vi "Generic_AR.vi"() -> ()   [LabVIEW 2018]
panel:
  in  "stop":bool
  out "Graph":u16[][](graph)
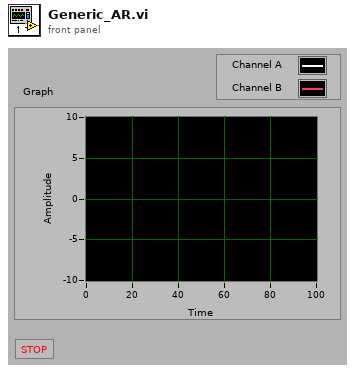
[diagram p1: front panel]
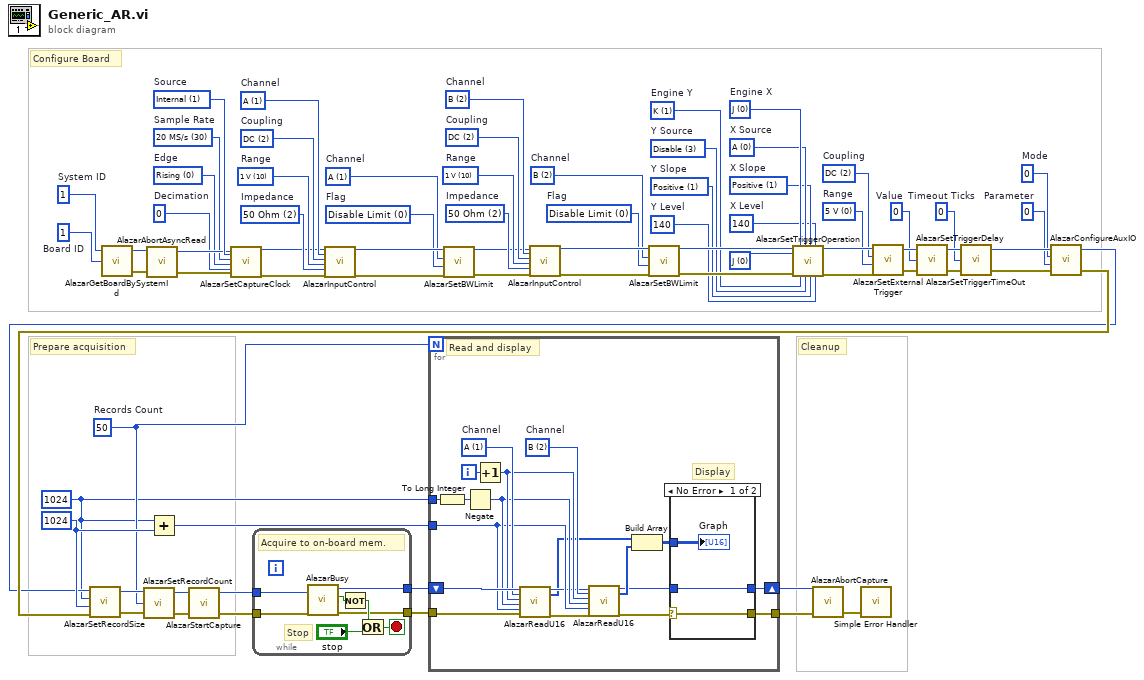
[diagram p0: block diagram]
diagram:
  w6 = u32 50  # Records Count
  w17 = u32 1024 ("Post-trigger Samples")
  w5 = u32 1024 ("Pre-trigger Samples")
  w47 = u32 0 items=["Disable Limit", "Enable Limit"]  # Flag
  w46 = u32 2 items=["A"=1, "B"=2, "C"=4, "D"=8]  # Channel
  w50 = u32 2 items=["1 MOhm"=1, "50 Ohm"=2]  # Impedance
  w44 = u32 10 items=["20 mV"=1, "40 mV"=2, "50 mV"=3, "80 mV"=4, "100 mV"=5, "200 mV"=6, "400 mV"=7, "500 mV"=8, "800 mV"=9, "1 V"=10, "1.25 V"=33, "2 V"=11, "4 V"=12, "5 V"=13, "8 V"=14, "10 V"=15, "20 V"=16]  # Range
  w51 = u32 2 items=["AC"=1, "DC"=2]  # Coupling
  w52 = u8 2 items=["A"=1, "B"=2, "C"=4, "D"=8]  # Channel
  w20 = u32 0  # Parameter
  w19 = u32 0  # Mode
  w18 = u32 0  # Timeout Ticks
  w25 = u32 0  # Value
  w29 = u32 0 items=["5 V", "1 V", "TTL"]  # Range
  w28 = u32 2 items=["AC"=1, "DC"=2]  # Coupling
  w32 = u32 140  # Y Level
  w33 = u32 1 items=["Positive"=1, "Negative"=2]  # Y Slope
  w34 = u32 3 items=["A", "B", "External", "Disable", "C", "D"]  # Y Source
  w36 = u32 140  # X Level
  w37 = u32 1 items=["Positive"=1, "Negative"=2]  # X Slope
  w38 = u32 0 items=["A", "B", "External", "Disable", "C", "D"]  # X Source
  w35 = u32 1 items=["J", "K"]  # Engine Y
  w39 = u32 0 items=["J", "K"]  # Engine X
  w40 = u32 0 items=["J", "K", "J OR K", "J AND K", "J XOR K", "J AND NOT K", "NOT J AND K"] ("Op.")
  w54 = u32 0 items=["Disable Limit", "Enable Limit"]  # Flag
  w53 = u32 1 items=["A"=1, "B"=2, "C"=4, "D"=8]  # Channel
  w59 = u32 2 items=["1 MOhm"=1, "50 Ohm"=2]  # Impedance
  w60 = u32 10 items=["20 mV"=1, "40 mV"=2, "50 mV"=3, "80 mV"=4, "100 mV"=5, "200 mV"=6, "400 mV"=7, "500 mV"=8, "800 mV"=9, "1 V"=10, "1.25 V"=33, "2 V"=11, "4 V"=12, "5 V"=13, "8 V"=14, "10 V"=15, "20 V"=16]  # Range
  w61 = u32 2 items=["AC"=1, "DC"=2]  # Coupling
  w62 = u8 1 items=["A"=1, "B"=2, "C"=4, "D"=8]  # Channel
  w64 = u32 0  # Decimation
  w65 = u32 0 items=["Rising", "Falling"]  # Edge
  w66 = u32 30 items=["1 kS/s"=1, "2 kS/s"=2, "5 kS/s"=4, "10 kS/s"=8, "20 kS/s"=10, "50 kS/s"=12, "100 kS/s"=14, "200 kS/s"=16, "500 kS/s"=18, "1 MS/s"=20, "2 MS/s"=24, "5 MS/s"=26, "10 MS/s"=28, "20 MS/s"=30, "25 MS/s"=33, "50 MS/s"=34, "100 MS/s"=36, "125 MS/s"=37, "160 MS/s"=38, "180 MS/s"=39, "250 MS/s"=43, "500 MS/s"=48, "800 MS/s"=50, "1000 MS/s"=53, "1200 MS/s"=55, "1500 MS/s"=58, "1800 MS/s"=61, "USER_DEF"=0]  # Sample Rate
  w68 = u32 1 items=["Internal"=1, "External"=2]  # Source
  w72 = u32 1  # Board ID
  w71 = u32 1  # System ID
  # "Cleanup"
  # "Prepare acquisition"
  # "Configure Board"
  n1 = call "AlazarGetBoardBySystemId.vi"("Board ID"=w72, "System ID"=w71) -> ("error out"=w69:errorcluster, "Handle"=w70:u64)  [unwired: 1 in, 1 out]
  n2 = call "AlazarAbortAsyncRead.vi"("Handle"=w70, "error in (no error)"=w69) -> ("Handle"=w67:u64, "error out"=w63:errorcluster)  [unwired: 1 out]
  n3 = Add(x=w5, y=w17) -> (x+y=w4:u32)
  n4 = call "AlazarSetCaptureClock.vi"("Handle"=w67, "Source"=w68, "Sample Rate"=w66, "Edge"=w65, "Decimation"=w64, "error in (no error)"=w63) -> ("Handle"=w58:u64, "error out"=w57:errorcluster)  [unwired: 11 in, 1 out]
  n5 = call "AlazarInputControl.vi"("Handle"=w58, "Channel"=w62, "Coupling"=w61, "Range"=w60, "Impedance"=w59, "error in (no error)"=w57) -> ("Handle"=w56:u64, "error out"=w55:errorcluster)  [unwired: 11 in, 1 out]
  n6 = call "AlazarSetBWLimit.vi"("error in (no error)"=w55, "Flag"=w54, "Channel"=w53, "Handle"=w56) -> ("error out"=w45:errorcluster, "Handle"=w43:u64)  [unwired: 1 out]
  n7 = call "AlazarInputControl.vi"("Handle"=w43, "Channel"=w52, "Coupling"=w51, "Range"=w44, "Impedance"=w50, "error in (no error)"=w45) -> ("Handle"=w49:u64, "error out"=w48:errorcluster)  [unwired: 11 in, 1 out]
  n8 = call "AlazarSetBWLimit.vi"("error in (no error)"=w48, "Flag"=w47, "Channel"=w46, "Handle"=w49) -> ("error out"=w41:errorcluster, "Handle"=w42:u64)  [unwired: 1 out]
  n9 = call "AlazarSetTriggerOperation.vi"("Handle"=w42, "Trigger Operation"=w40, "error in (no error)"=w41, "Trigger Engine 1"=w39, "Trigger Engine 2"=w35, "Source 1"=w38, "Source 2"=w34, "Slope 1"=w37, "Slope 2"=w33, "Level 1"=w36, "Level 2"=w32) -> ("Handle"=w31:u64, "error out"=w30:errorcluster)  [unwired: 6 in, 1 out]
  n10 = call "AlazarSetExternalTrigger.vi"("error in (no error)"=w30, "Range ID"=w29, "Coupling ID"=w28, "Handle"=w31) -> ("error out"=w26:errorcluster, "Handle"=w27:u64)  [unwired: 1 out]
  n11 = call "AlazarSetTriggerDelay.vi"("error in (no error)"=w26, "Delay"=w25, "Handle"=w27) -> ("error out"=w23:errorcluster, "Handle"=w24:u64)  [unwired: 1 out]
  n12 = call "AlazarSetTriggerTimeOut.vi"("error in (no error)"=w23, "Timeout Ticks"=w18, "Handle"=w24) -> ("error out"=w21:errorcluster, "Handle"=w22:u64)  [unwired: 1 out]
  n13 = call "AlazarConfigureAuxIO.vi"("error in (no error)"=w21, "Parameter"=w20, "Mode"=w19, "Handle"=w22) -> ("error out"=w16:errorcluster, "Handle"=w15:u64)  [unwired: 1 out]
  n14 = call "AlazarSetRecordSize.vi"("error in (no error)"=w16, "Post-trigger Samples"=w17, "Pre-trigger Samples"=w5, "Handle"=w15) -> ("error out"=w13:errorcluster, "Handle"=w14:u64)  [unwired: 1 out]
  n15 = call "AlazarSetRecordCount.vi"("error in (no error)"=w13, "Count"=w6, "Handle"=w14) -> ("error out"=w11:errorcluster, "Handle"=w12:u64)  [unwired: 1 out]
  n16 = call "AlazarStartCapture.vi"("Handle"=w12, "error in (no error)"=w11) -> ("Handle"=w10:u64, "error out"=w9:errorcluster)  [unwired: 1 out]
  n17 = while {
    tunnel: w10 -> [w77]
    tunnel: w9 -> [w76]
    tunnel: [w75] -> w8
    tunnel: [w74] -> w7
    stop <- w80 stop-if-true
    # "Stop"
    # "Acquire to on-board mem."
    n18 = call "AlazarBusy.vi"("Handle"=w77, "error in (no error)"=w76) -> ("Handle"=w75:u64, "Busy"=w79:bool, "error out"=w74:errorcluster)  [unwired: 1 out]
    n19 = Not(x=w79) -> (.not. x?=w78:bool)
    n20 = Or(x=w78, y="stop") -> (x .or. y?=w80:bool)
  }
  n21 = for {
    N: w6 -> [_]
    tunnel: [w93] -> w3
    shift-right: [w81] -> w2
    shift-left: w8 -> [w99]
    tunnel: w7 -> [w98]
    tunnel: w5 -> [w95]
    tunnel: w4 -> [w89]
    i -> [w96]
    w92 = u32 2 items=["B"=2]  # Channel
    w97 = u32 1 items=["A"=1]  # Channel
    # "Read and display"
    # "Display"
    n22 = To Long Integer(number=w95) -> (32bit integer=w94:i32)
    n23 = Negate(x=w94) -> (-x=w90:i32)
    n24 = Increment(x=w96) -> (x+1=w91:i32)
    n25 = call "AlazarReadU16.vi"("Handle"=w99, "Channel"=w97, "Record"=w91, "Transfer Offset"=w90, "Transfer Length"=w89, "error in (no error)"=w98) -> ("Handle"=w88:u64, "Buffer"=w86:u16[], "error out"=w87:errorcluster)  [unwired: 10 in, 1 out]
    n26 = call "AlazarReadU16.vi"("Handle"=w88, "Channel"=w92, "Record"=w91, "Transfer Offset"=w90, "Transfer Length"=w89, "error in (no error)"=w87) -> ("Handle"=w82:u64, "Buffer"=w85:u16[], "error out"=w83:errorcluster)  [unwired: 10 in, 1 out]
    n27 = Build Array(w86, w85) -> (w84:u16[][])
    n28 = case shown="No Error" w83 {
      selector: w83 -> [w102 w104]
      tunnel: [w102 w104] -> w93
      tunnel: w84 -> [w101 _]
      tunnel: w82 -> [w100 w103]
      tunnel: [w100 w103] -> w81
      frame No Error {
        "Graph" <- w101
      }
      frame Error {
      }
    }
  }
  n29 = call "AlazarAbortCapture.vi"("Handle"=w2, "error in (no error)"=w3) -> ("error out"=w1:errorcluster)  [unwired: 2 out]
  n30 = call <vilib>:"Simple Error Handler.vi"("error in (no error)"=w1) -> ()  [unwired: 4 in, 5 out]
